vi "Default.File.Add Line to Text Log File.vi"   [LabVIEW 2010]
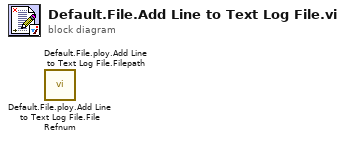
[diagram p0: block diagram]
diagram:
  n1 = call "Default.File.ploy.Add Line to Text Log File.File Refnum.vi"() -> ()  [unwired: 10 in, 2 out]
  n2 = call "Default.File.ploy.Add Line to Text Log File.Filepath.vi"() -> ()  [unwired: 10 in, 2 out]
